vi "Convergence Study (Trap vs. Simp).vi"() -> ()   [LabVIEW 2017]
uses:
  <vilib>/Analysis/8numeric.llb/1D Numeric Integration.vi
  <vilib>/Analysis/NI_AALPro.lvlib
panel:
  in  "Digitizing Parameters":T1={"Number of Samples"=100, "Lower Limit"=0.0, "Upper Limit"=1.0}
  in  "Function Parameters":cluster{"Prefactor":dbl, "Power":dbl}={"Prefactor"=5.0, "Power"=4.0}
  out "XY Graph":cluster{i32[], dbl[]}[](graph)
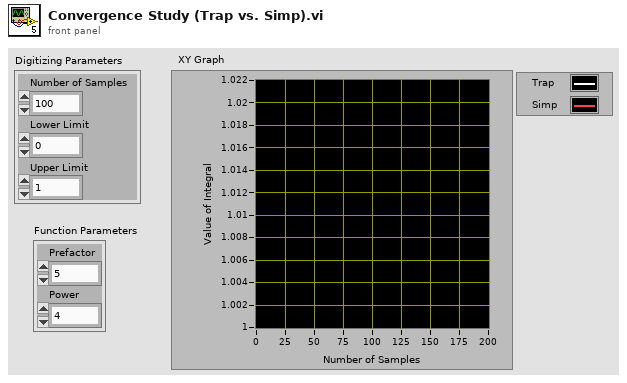
[diagram p1: front panel]
types:
  T1 = cluster{"Number of Samples":i32, "Lower Limit":dbl, "Upper Limit":dbl}
  T2 = cluster{"X Array":dbl[], "Y Array":dbl[], "delta_x":dbl}
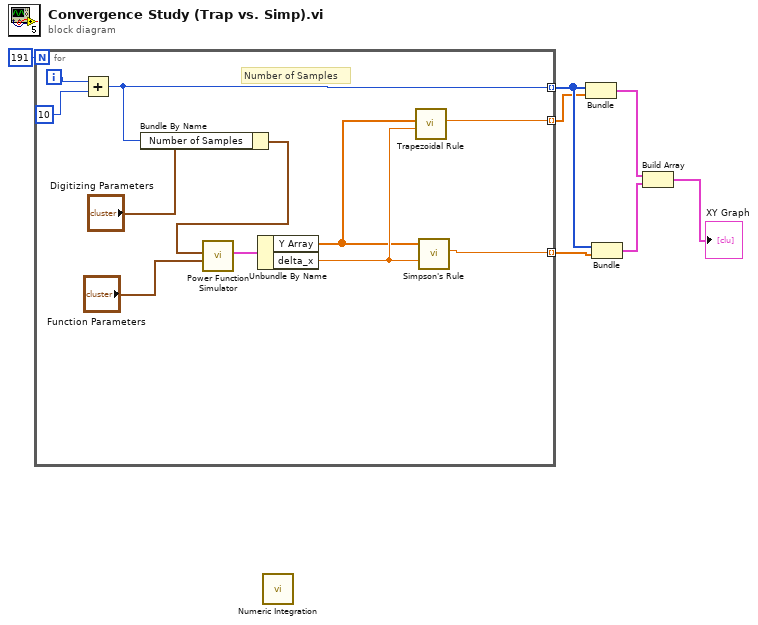
[diagram p0: block diagram]
diagram:
  n1 = for {
    N: 191 -> [_]
    tunnel: [w9] -> w6 mode=indexing
    tunnel: [w12] -> w5 mode=indexing
    tunnel: [w11] -> w4 mode=indexing
    i -> [w14]
    # "Number of Samples"
    n2 = Add(x=w14, y=10) -> (x+y=w9:i32)
    n3 = Bundle By Name(cluster="Digitizing Parameters", "Number of Samples"=w9) -> (w8:T1)
    n4 = call "Power Function Simulator.vi"("Function Parameters"="Function Parameters", "Digitizing Parameters"=w8) -> ("Output Cluster"=w17:T2)  [unwired: 9 in]
    n5 = Unbundle By Name(w17) -> ("Y Array"=w15:dbl[], "delta_x"=w16:dbl)
    n6 = call "Trapezoidal Rule.vi"("Delta_x"=w16, "y array"=w15) -> ("Value of Integral"=w12:dbl)  [unwired: 9 in]
    n7 = call "Simpson's Rule.vi"("delta_x"=w16, "Array"=w15) -> ("Value of Integral"=w11:dbl)  [unwired: 9 in]
  }
  n8 = call-poly <vilib>:"Numeric Integration.vi"() -> ()  [unwired: 3 in, 2 out]
  n9 = Bundle(w6, w5) -> (w3:cluster{i32[], dbl[]})  [unwired: 1 in]
  n10 = Bundle(w6, w4) -> (w2:cluster{i32[], dbl[]})  [unwired: 1 in]
  n11 = Build Array(w3, w2) -> (→"XY Graph":cluster{i32[], dbl[]}[])
